vi "Countertask2.vi"(8 "error in":errorcluster caption="错误输入") -> (0 "error out":errorcluster caption="错误输出", 3 "task out":refnum<k21> caption="任务输出")   [LabVIEW 2020]
uses:
  <vilib>/DAQmx/create/channels.llb/DAQmx Create Channel (CI-Position-Angular Encoder).vi
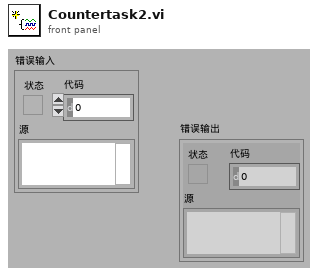
[diagram p1: front panel]
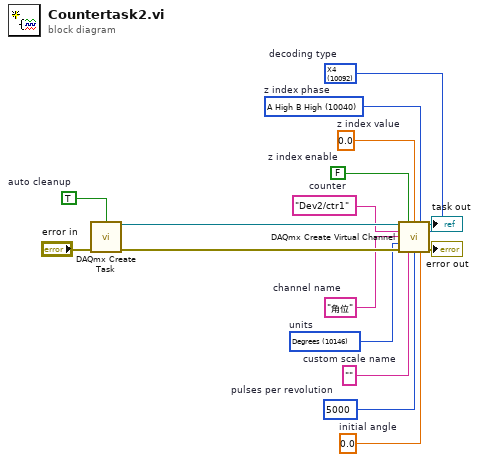
[diagram p0: block diagram]
diagram:
  w5 = 10146 items=["Degrees"=10146, "Radians"=10273, "Ticks"=10304, "From Custom Scale"=10065]  # units
  w1 = 10092 items=["X1"=10090, "X2"=10091, "X4"=10092, "Two Pulse Counting"=10313]  # decoding type
  w2 = 0.0  # initial angle
  w3 = u32 5000  # pulses per revolution
  w4 = ""  # custom scale name
  w6 = 10040 items=["A High B High"=10040, "A High B Low"=10041, "A Low B High"=10042, "A Low B Low"=10043]  # z index phase
  w7 = 0.0  # z index value
  w8 = FALSE  # z index enable
  w9 = "角位"  # channel name
  w12 = "Dev2/ctr1"  # counter
  w14 = TRUE  # auto cleanup
  n1 = call <vilib>:"DAQmx Create Task.vi"("auto cleanup"=w14, "error in"="error in") -> ("task out"=w13:refnum<k21>, "error out"=w15:errorcluster)  [unwired: 12 in]
  n2 = call-poly <vilib>:"DAQmx Create Virtual Channel.vi"("task in"=w13, "z index enable"=w8, "z index value"=w7, "z index phase"=w6, "counter"=w12, "decoding type"=w1, "name to assign"=w9, "units"=w5, "error in"=w15, "custom scale name"=w4, "pulses per revolution"=w3, "initial angle"=w2) -> ("task out"=→"task out":refnum<k21>, "error out"=→"error out":errorcluster)  [unwired: 2 in]
